vi "interpolate nodes.vi"(10 "Interpolate spacing":dbl format="%#_6pm", 11 "Nodes on the line\n(  x      ,       y   )":dbl[][](array[numeric])=[[-5e-06, -5e-06], [5e-06, 5e-06]] min=-4.5e-05 max=4.5e-05 step=1e-09 format="%#_6pm") -> (3 "Interpolate result":dbl[][](array[numeric]))   [LabVIEW 2013]
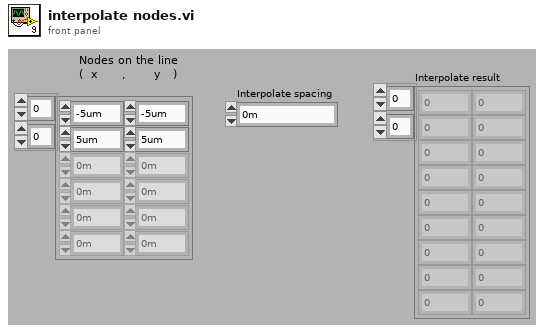
[diagram p1: front panel]
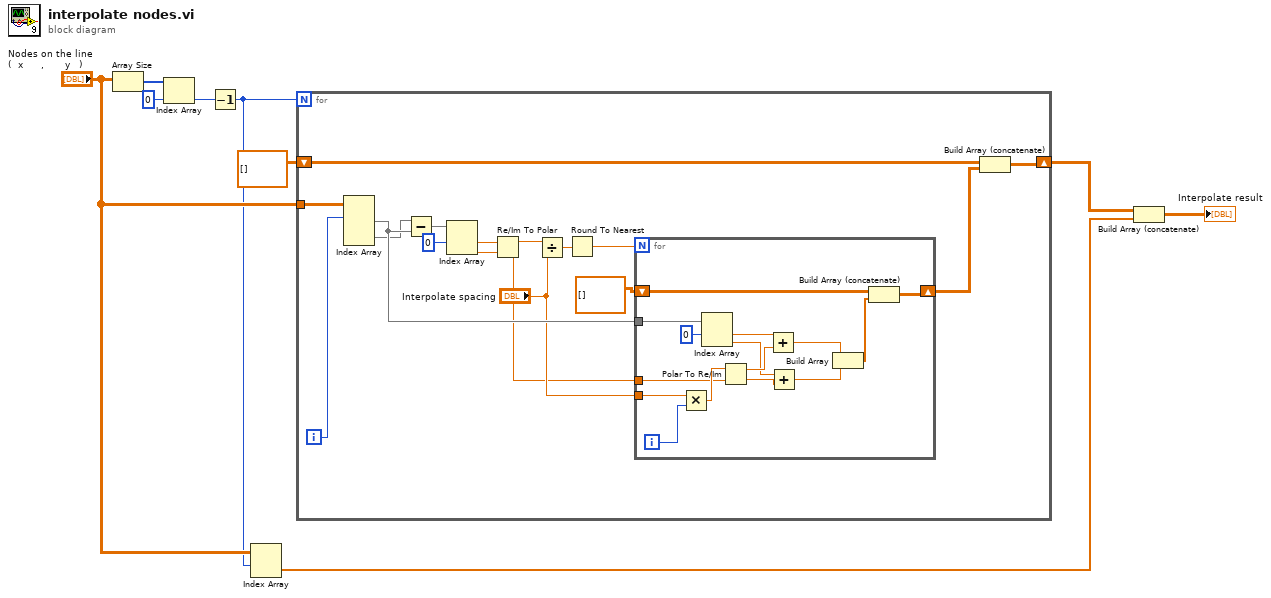
[diagram p0: block diagram]
diagram:
  n1 = Array Size(array="Nodes on the line\n(  x      ,       y   )") -> (size(s)=w9:i32[])
  n2 = Index Array(array=w9, index=0) -> (element=w5:i32)
  n3 = Decrement(x=w5) -> (x-1=w1:i32)
  n4 = Index Array(array="Nodes on the line\n(  x      ,       y   )", index (row)=w1) -> (element=w3:dbl[])  [unwired: 1 in]
  n5 = for {
    N: w1 -> [_]
    tunnel: "Nodes on the line\n(  x      ,       y   )" -> [w26]
    shift-right: [w12] -> w4
    shift-left: dbl[][] [] -> [w11]
    i -> [w25]
    n6 = Index Array(array=w26, index (row) #1=w25) -> (element #1=w18:dbl[], element #2=w14:dbl[])  [unwired: 3 in]
    n7 = Subtract(x=w14, y=w18) -> (x-y=w24:dbl[])
    n8 = Index Array(array=w24, index #1=0 ("index")) -> (element #1=w22:dbl, element #2=w21:dbl)  [unwired: 1 in]
    n9 = Re/Im To Polar(2:w21, 3:w22) -> (0:w16:dbl, 1:w20:dbl)
    n10 = Divide(x=w20, y="Interpolate spacing") -> (x/y=w19:dbl)
    n11 = Round To Nearest(number=w19) -> (nearest integer value=w10:dbl)
    n12 = for {
      N: w10 -> [_]
      tunnel: w18 -> [w37]
      tunnel: "Interpolate spacing" -> [w41]
      tunnel: w16 -> [w38]
      shift-right: [w28] -> w13
      shift-left: dbl[][] [] -> [w27]
      i -> [w40]
      n13 = Multiply(x=w41, y=w40) -> (x*y=w39:dbl)
      n14 = Index Array(array=w37, index #1=0 ("index")) -> (element #1=w35:dbl, element #2=w33:dbl)  [unwired: 1 in]
      n15 = Polar To Re/Im(2:w38, 3:w39) -> (0:w32:dbl, 1:w34:dbl)
      n16 = Add(x=w35, y=w34) -> (x+y=w31:dbl)
      n17 = Add(x=w33, y=w32) -> (x+y=w30:dbl)
      n18 = Build Array(w31, w30) -> (w29:dbl[])
      n19 = Build Array (concatenate)(w27, w29) -> (w28:dbl[][])
    }
    n20 = Build Array (concatenate)(w11, w13) -> (w12:dbl[][])
  }
  n21 = Build Array (concatenate)(w4, w3) -> (→"Interpolate result":dbl[][])
